vi "in_delta values.vi"(11 "x array":dbl[](array[numeric])) -> (3 "x delta values":dbl[](array[numeric]))   [LabVIEW 2017, in "NI_Gmath.lvlib"]
uses:
  <vilib>/gmath/NI_Gmath.lvlib
  <vilib>/Analysis/2dsp.llb/Derivative x(t).vi
  <vilib>/Analysis/NI_AALPro.lvlib
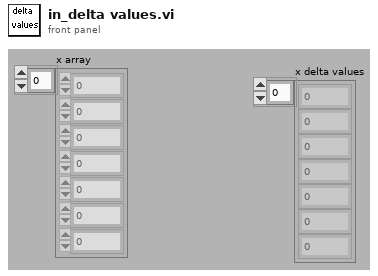
[diagram p1: front panel]
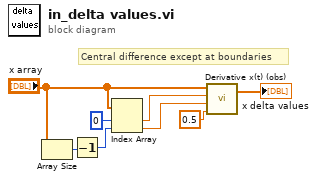
[diagram p0: block diagram]
diagram:
  # "Central difference except at boundaries"
  n1 = Array Size(array="x array") -> (size(s)=w7:i32)
  n2 = Decrement(x=w7) -> (x-1=w1:i32)
  n3 = Index Array(array="x array", index #1=0 ("index"), index #2=w1) -> (element #1=w4:dbl, element #2=w3:dbl)
  n4 = call <vilib>:"Derivative x(t) (obs).vi"("dt"=0.5, "final condition"=w3, "initial condition"=w4, "X"="x array") -> ("dX/dt"=→"x delta values":dbl[])  [unwired: 1 out]
